vi "TIFFStream Open.vi"(6 "Bytes per strip":u32=8000, 7 "File path":path, 8 "error in (no error)":errorcluster, 9 "Height Pixels":u32, 10 "Width Pixels":u32, 11 "Big endian?":bool) -> (0 "error out":errorcluster, 1 "Next IFD Offset":u32, 2 "Image data reference":refnum<data-value>, 3 "File data":T1)   [LabVIEW 2015]
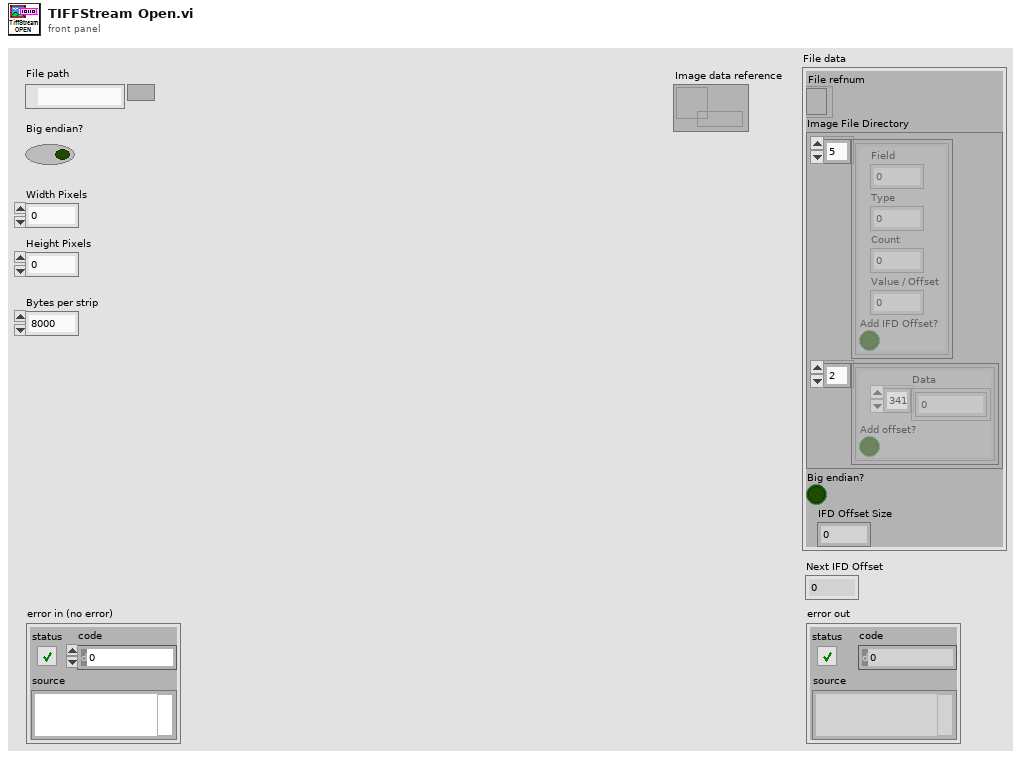
[diagram p1: front panel]
types:
  T1 = cluster{"File refnum":refnum<file>, "Image File Directory":cluster{cluster{"Field":u16, "Type":u16, "Count":u32, "Value / Offset":u32, "Add IFD Offset?":bool}[], cluster{"Data":u32[], "Add offset?":bool}[]}, "Big endian?":bool, "IFD Offset Size":u32}
  T2 = cluster{"Field":u16, "Type":u16, "Count":u32, "Value / Offset":u32, "Add IFD Offset?":bool}
  T3 = enum16{"big-endian, network order", "native, host order", "little-endian"}
  T4 = enum16{"open", "replace", "create", "open or create", "replace or create", "replace or create with confirmation"}
  T5 = cluster{"Field":u16, "Type":u16, "Count":u32, "Value / Offset":u32, "Add IFD Offset?":bool}[]
  T6 = cluster{cluster{"Field":u16, "Type":u16, "Count":u32, "Value / Offset":u32, "Add IFD Offset?":bool}[], cluster{"Data":u32[], "Add offset?":bool}[]}
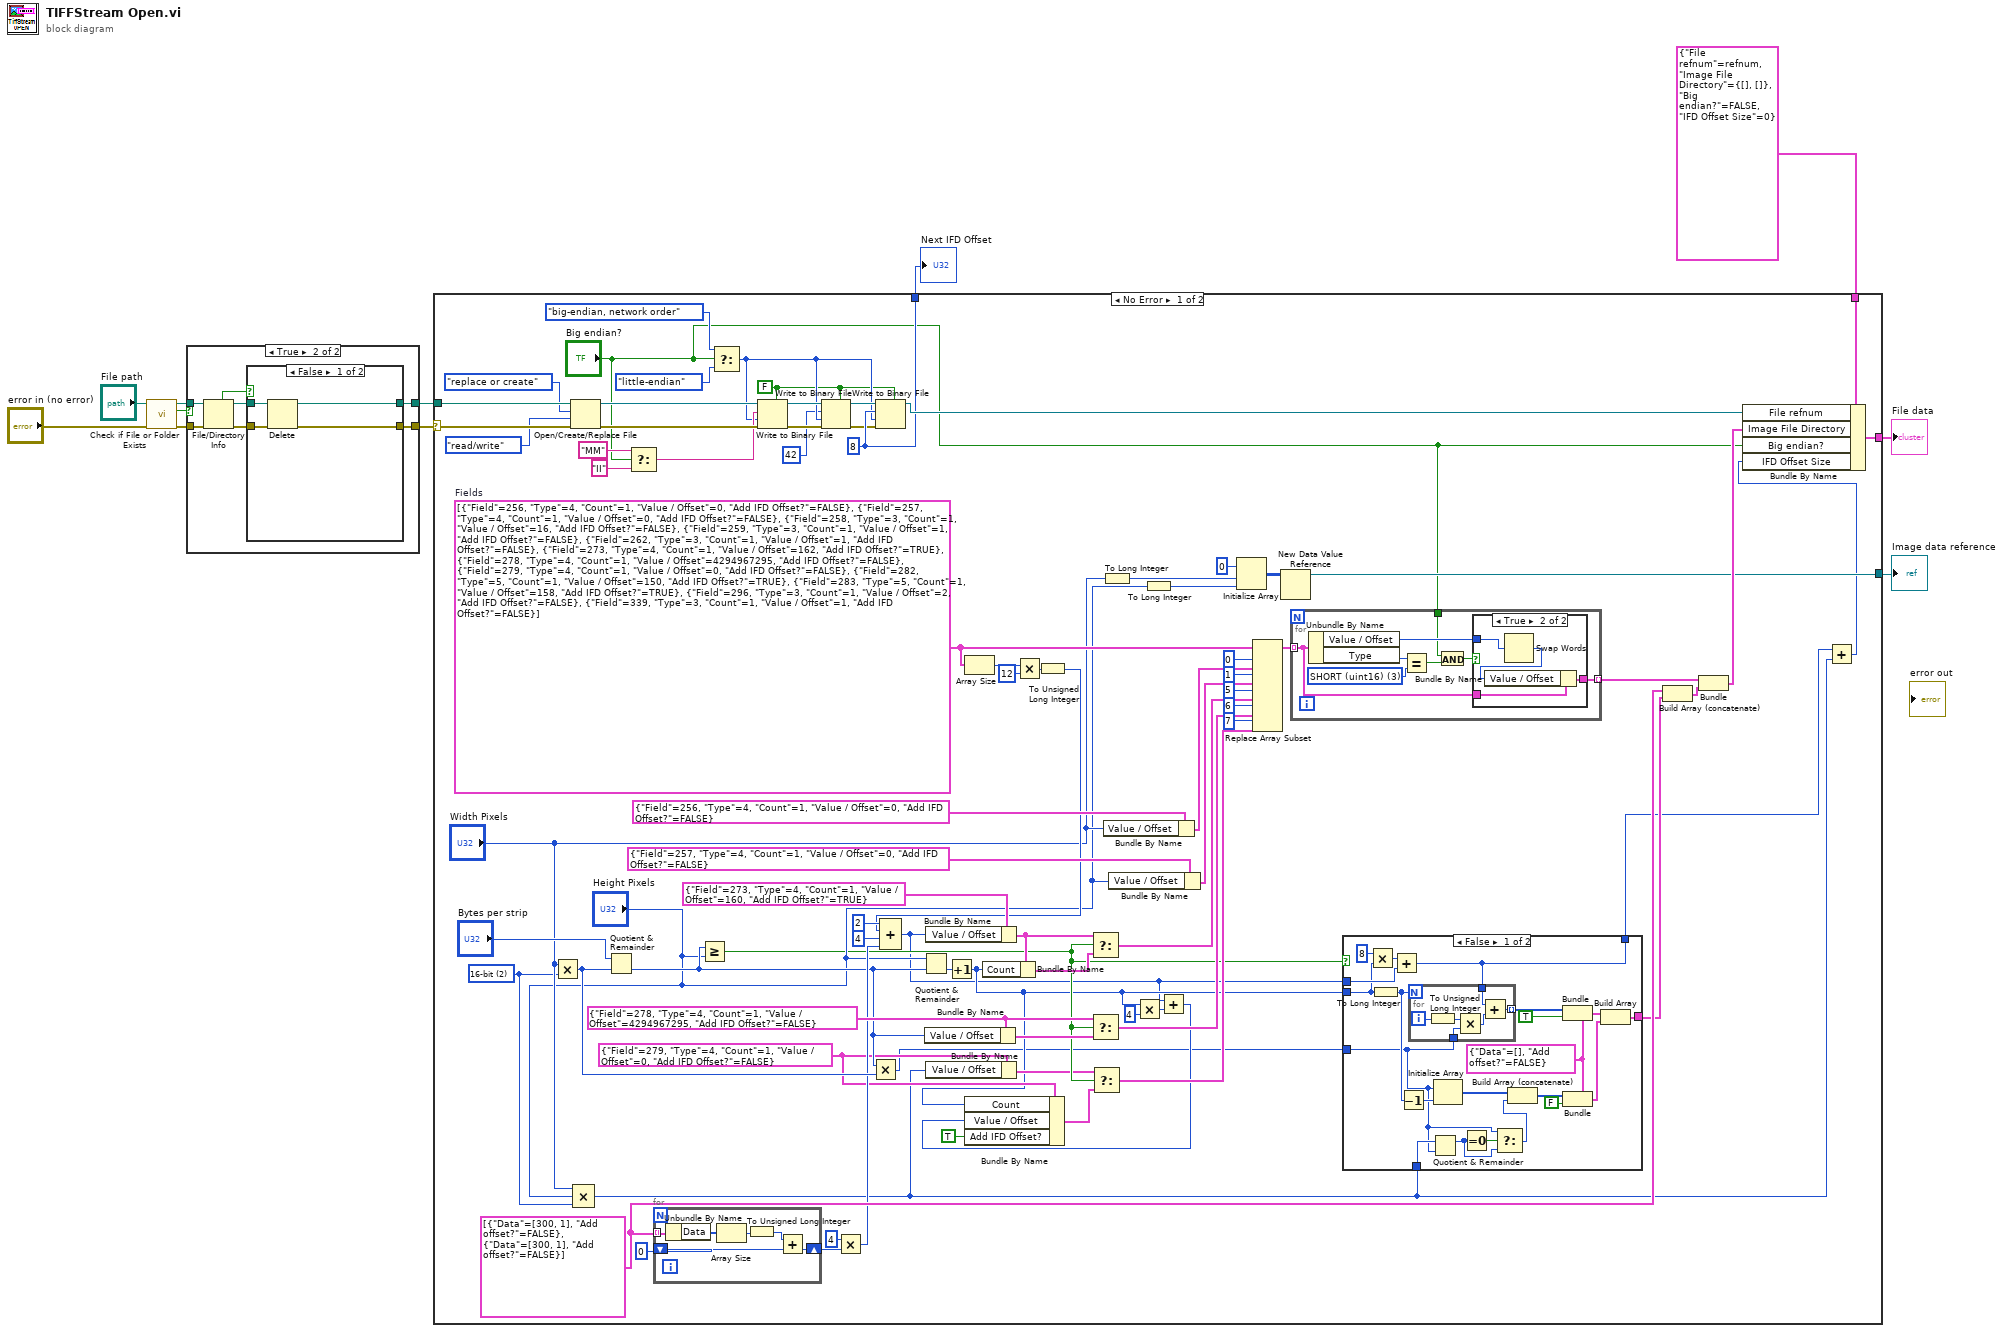
[diagram p0: block diagram]
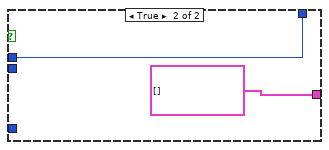
[diagram p3: hidden frame]
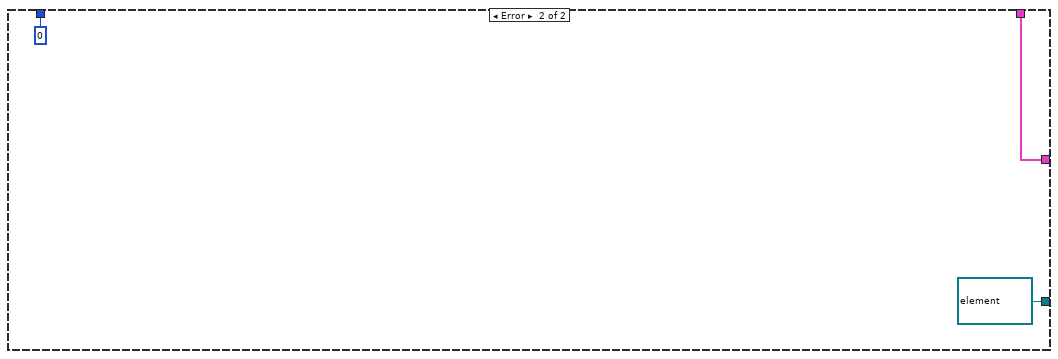
[diagram p4: hidden frame]
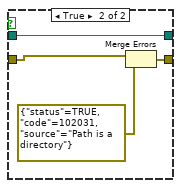
[diagram p6: hidden frame]
diagram:
  n1 = call <vilib>:"Check if File or Folder Exists.vi"("error in (no error)"="error in (no error)", "path"="File path") -> ("error out"=w9:errorcluster, "file or folder exists?"=w10:bool, "dup path"=w8:path)  [unwired: 7 in]
  n2 = case shown="True" w10 {
    tunnel: w9 -> [w13 w19]
    tunnel: w8 -> [w12 w17]
    tunnel: [w13 w20] -> w6
    tunnel: [w12 w14] -> w5
    frame False {
    }
    frame True {
      n3 = File/Directory Info(path=w17, error in=w19) -> (path out=w15:path, directory=w16:bool, error out=w18:errorcluster)  [unwired: 4 out]
      n4 = case shown="False" w16 {
        tunnel: [w24 w26] -> w20
        tunnel: w18 -> [w23 w28]
        tunnel: w15 -> [w22 w27]
        tunnel: [w21 w27] -> w14
        frame False {
          n5 = Delete(path (use dialog)=w22, error in=w23) -> (deleted path=w21:path, error out=w24:errorcluster)  [unwired: 3 in, 1 out]
        }
        frame True {
          n6 = Merge Errors(w28, errorcluster {"status"=TRUE, "code"=102031, "source"="Path is a directory"} ("error in")) -> (w26:errorcluster)
        }
      }
    }
  }
  n7 = case shown="No Error" w6 {
    selector: w6 -> [w110 _]
    tunnel: w5 -> [w111 _]
    tunnel: [w100 w162] -> w3
    tunnel: T1 {"File refnum"=refnum, "Image File Directory"={[], []}, "Big endian?"=FALSE, "IFD Offset Size"=0} ("File data") -> [w101 w162]
    tunnel: [w77 u32 0] -> w2
    tunnel: [w74 refnum<data-value> refnum ("data value reference")] -> w1
    frame No Error {
      w39 = T2 {"Field"=279, "Type"=4, "Count"=1, "Value / Offset"=0, "Add IFD Offset?"=FALSE}
      w44 = u32 2 items=["8-bit"=1, "16-bit"=2, "32-bit"=4, "64-bit"=8]
      w80 = T2 {"Field"=278, "Type"=4, "Count"=1, "Value / Offset"=4294967295, "Add IFD Offset?"=FALSE}
      w71 = cluster{"Data":u32[], "Add offset?":bool}[] [{"Data"=[300, 1], "Add offset?"=FALSE}, {"Data"=[300, 1], "Add offset?"=FALSE}]
      w72 = T5 [{"Field"=256, "Type"=4, "Count"=1, "Value / Offset"=0, "Add IFD Offset?"=FALSE}, {"Field"=257, "Type"=4, "Count"=1, "Value / Offset"=0, "Add IFD Offset?"=FALSE}, {"Field"=258, "Type"=3, "Count"=1, "Value / Offset"=16, "Add IFD Offset?"=FALSE}, {"Field"=259, "Type"=3, "Count"=1, "Value / Offset"=1, "Add IFD Offset?"=FALSE}, {"Field"=262, "Type"=3, "Count"=1, "Value / Offset"=1, "Add IFD Offset?"=FALSE}, {"Field"=273, "Type"=4, "Count"=1, "Value / Offset"=162, "Add IFD Offset?"=TRUE}, {"Field"=278, "Type"=4, "Count"=1, "Value / Offset"=4294967295, "Add IFD Offset?"=FALSE}, {"Field"=279, "Type"=4, "Count"=1, "Value / Offset"=0, "Add IFD Offset?"=FALSE}, {"Field"=282, "Type"=5, "Count"=1, "Value / Offset"=150, "Add IFD Offset?"=TRUE}, {"Field"=283, "Type"=5, "Count"=1, "Value / Offset"=158, "Add IFD Offset?"=TRUE}, {"Field"=296, "Type"=3, "Count"=1, "Value / Offset"=2, "Add IFD Offset?"=FALSE}, {"Field"=339, "Type"=3, "Count"=1, "Value / Offset"=1, "Add IFD Offset?"=FALSE}]  # Fields
      w77 = u32 8
      w56 = FALSE ("prepend array or string size? (T)")
      n8 = Multiply(x="Width Pixels", y=w44) -> (x*y=w64:u32)
      n9 = Open/Create/Replace File(file path (use dialog)=w111, error in=w110, operation (0:open)=T4."replace or create", access (0:read/write)=enum16{"read/write", "read-only", "write-only"}."read/write") -> (refnum out=w107:refnum<file>, error out=w104:errorcluster)  [unwired: 2 in, 1 out]
      n10 = Compound Arithmetic op=MULTIPLY("Width Pixels", "Height Pixels", w44) -> (w30:u32)
      n11 = Quotient & Remainder(x="Bytes per strip", y=w64) -> (floor(x/y)=w47:u32)  [unwired: 1 out]
      n12 = Select(t="MM", s="Big endian?", f="II") -> (s? t:f=w62:string)
      n13 = for {
        tunnel: w71 -> [w159] mode=indexing
        shift-right: [w156] -> w69
        shift-left: u32 0 -> [w155]
        n14 = Unbundle By Name(w159) -> ("Data"=w158:u32[])
        n15 = Array Size(array=w158) -> (size(s)=w157:i32)
        n16 = To Unsigned Long Integer(number=w157) -> (unsigned 32bit integer=w154:u32)
        n17 = Add(x=w154, y=w155) -> (x+y=w156:u32)
      }
      n18 = Greater Or Equal?(x=w47, y="Height Pixels") -> (x >= y?=w41:bool)
      n19 = Select(t=T3."big-endian, network order" ("byte order (0:big-endian, network order)"), s="Big endian?", f=T3."little-endian") -> (s? t:f=w57:T3)
      n20 = Write to Binary File(file (use dialog)=w107, data=w62, error in=w104, 5:w56, 9:w57) -> (refnum out=w59:refnum<file>, error out=w61:errorcluster)  [unwired: 1 in, 1 out]
      n21 = Write to Binary File(file (use dialog)=w59, data=u16 42, error in=w61, 5:w56, 9:w57) -> (refnum out=w58:refnum<file>, error out=w60:errorcluster)  [unwired: 1 in, 1 out]
      n22 = Multiply(x=u32 4, y=w69) -> (x*y=w52:u32)
      n23 = Multiply(x=w47, y=w64) -> (x*y=w31:u32)
      n24 = Write to Binary File(file (use dialog)=w58, data=w77, error in=w60, 5:w56, 9:w57) -> (refnum out=w99:refnum<file>)  [unwired: 1 in, 2 out]
      n25 = Quotient & Remainder(x="Height Pixels", y=w47) -> (floor(x/y)=w48:u32)  [unwired: 1 out]
      n26 = Bundle By Name(cluster=w80, "Value / Offset"=w47) -> (w79:T2)
      n27 = Bundle By Name(cluster=w39, "Value / Offset"=w30) -> (w40:T2)
      n28 = Increment(x=w48) -> (x+1=w34:u32)
      n29 = Array Size(array=w72) -> (size(s)=w96:i32)
      n30 = Multiply(x=w96, y=12) -> (x*y=w97:i32)
      n31 = To Unsigned Long Integer(number=w97) -> (unsigned 32bit integer=w50:u32)
      n32 = Compound Arithmetic op=ADD(u32 2 ("value"), w50, u32 4 ("value"), w52) -> (w33:u32)
      n33 = Bundle By Name(cluster=T2 {"Field"=273, "Type"=4, "Count"=1, "Value / Offset"=160, "Add IFD Offset?"=TRUE}, "Value / Offset"=w33) -> (w73:T2)
      n34 = Bundle By Name(cluster=w73, "Count"=w34) -> (w85:T2)
      n35 = Select(t=w73, s=w41, f=w85) -> (s? t:f=w82:T2)
      n36 = Select(t=w80, s=w41, f=w79) -> (s? t:f=w81:T2)
      n37 = To Long Integer(number="Width Pixels") -> (32bit integer=w68:i32)
      n38 = Bundle By Name(cluster=T2 {"Field"=256, "Type"=4, "Count"=1, "Value / Offset"=0, "Add IFD Offset?"=FALSE}, "Value / Offset"="Width Pixels") -> (w90:T2)
      n39 = Bundle By Name(cluster=T2 {"Field"=257, "Type"=4, "Count"=1, "Value / Offset"=0, "Add IFD Offset?"=FALSE}, "Value / Offset"="Height Pixels") -> (w89:T2)
      n40 = Multiply(x=w34, y=u32 4 ("x")) -> (x*y=w36:u32)
      n41 = To Long Integer(number="Height Pixels") -> (32bit integer=w67:i32)
      n42 = Add(x=w33, y=w36) -> (x+y=w32:u32)
      n43 = Bundle By Name(cluster=w39, "Count"=w34, "Value / Offset"=w32, "Add IFD Offset?"=TRUE) -> (w38:T2)
      n44 = Select(t=w40, s=w41, f=w38) -> (s? t:f=w42:T2)
      n45 = Initialize Array(u16 0 ("element"), w68, w67) -> (w75:u16[][])
      n46 = Replace Array Subset(array=w72, new element #1=w90, index #1=0 ("index"), new element #2=w89, index #2=1 ("index"), new element #3=w82, index #3=5 ("index"), new element #4=w81, index #4=6 ("index"), new element #5=w42, index #5=7 ("index")) -> (w54:T5)
      n47 = New Data Value Reference(data value=w75) -> (data value reference=w74:refnum<data-value>)  [unwired: 1 in, 1 out]
      n48 = for {
        tunnel: w54 -> [w116] mode=indexing
        tunnel: [w115] -> w53 mode=indexing
        tunnel: "Big endian?" -> [w112]
        w119 = u16 3 items=["BYTE (uint8)"=1, "ASCII"=2, "SHORT (uint16)"=3, "LONG (uint32)"=4, "RATIONAL (2 x LONG)"=5, "SBYTE (int8)"=6, "UNDEFINED"=7, "SSHORT (int16)"=8, "SLONG (int32)"=9, "SRATIONAL (2 x SLONG)"=10, "FLOAT"=11, "DOUBLE"=12] ("Type")
        n49 = Unbundle By Name(w116) -> ("Value / Offset"=w117:u32, "Type"=w118:u16)
        n50 = Equal?(x=w118, y=w119) -> (x = y?=w113:bool)
        n51 = And(x=w112, y=w113) -> (x .and. y?=w114:bool)
        n52 = case shown="True" w114 {
          tunnel: w117 -> [_ w122]
          tunnel: w116 -> [w120 w124]
          tunnel: [w120 w123] -> w115
          frame False {
          }
          frame True {
            n53 = Swap Words(1:w122) -> (0:w121:u32)
            n54 = Bundle By Name(cluster=w124, "Value / Offset"=w121) -> (w123:T2)
          }
        }
      }
      n55 = case shown="False" w41 {
        tunnel: w34 -> [w135 _]
        tunnel: [w142 cluster{"Data":u32[], "Add offset?":bool}[] []] -> w70
        tunnel: w31 -> [w126 _]
        tunnel: w33 -> [w139 w152]
        tunnel: [w138 w152] -> w37
        tunnel: w30 -> [w130 _]
        frame False {
          w137 = cluster{"Data":u32[], "Add offset?":bool} {"Data"=[], "Add offset?"=FALSE}
          n56 = Multiply(x=u32 8, y=w135) -> (x*y=w141:u32)
          n57 = To Long Integer(number=w135) -> (32bit integer=w134:i32)
          n58 = Add(x=w141, y=w139) -> (x+y=w138:u32)
          n59 = Decrement(x=w134) -> (x-1=w136:i32)
          n60 = for {
            N: w134 -> [_]
            tunnel: [w150] -> w145 mode=indexing
            tunnel: w138 -> [w149]
            tunnel: w126 -> [w146]
            i -> [w151]
            n61 = To Unsigned Long Integer(number=w151) -> (unsigned 32bit integer=w148:u32)
            n62 = Multiply(x=w148, y=w146) -> (x*y=w147:u32)
            n63 = Add(x=w149, y=w147) -> (x+y=w150:u32)
          }
          n64 = Quotient & Remainder(x=w130, y=w126) -> (x-y*floor(x/y)=w127:u32)  [unwired: 1 out]
          n65 = Initialize Array(w126, w136) -> (w132:u32[])
          n66 = Equal To 0?(x=w127) -> (x = 0?=w128:bool)
          n67 = Select(t=w126, s=w128, f=w127) -> (s? t:f=w125:u32)
          n68 = Build Array (concatenate)(w132, w125) -> (w131:u32[])
          n69 = Bundle(cluster=w137, "Data"=w145, "Add offset?"=TRUE) -> (w143:cluster{"Data":u32[], "Add offset?":bool})
          n70 = Bundle(cluster=w137, "Data"=w131, "Add offset?"=FALSE) -> (w129:cluster{"Data":u32[], "Add offset?":bool})
          n71 = Build Array(w143, w129) -> (w142:cluster{"Data":u32[], "Add offset?":bool}[])
        }
        frame True {
        }
      }
      n72 = Build Array (concatenate)(w71, w70) -> (w78:cluster{"Data":u32[], "Add offset?":bool}[])
      n73 = Bundle(w53, w78) -> (w98:T6)  [unwired: 1 in]
      n74 = Add(x=w37, y=w30) -> (x+y=w46:u32)
      n75 = Bundle By Name(cluster=w101, "File refnum"=w99, "Image File Directory"=w98, "Big endian?"="Big endian?", "IFD Offset Size"=w46) -> (w100:T1)
    }
    frame Error {
    }
  }
  "Next IFD Offset" <- w2
  "File data" <- w3
  "Image data reference" <- w1
